vi "Create from SCP Receive.vi"(8 "Error In":errorcluster, 10 "Remote Source Path":string, 11 "Session":refnum<class "Session.lvclass">) -> (0 "Error Out":errorcluster, 2 "File Information":T3, 3 "Channel":refnum<class "Channel.lvclass">)   [LabVIEW 2021, in "Field_RnD_Services_LIBSSH2_Toolkit.lvlib" / "Channel.lvclass"]
doc: "Creates a new Channel object from a Session object but configured for downloading a file from a remote SSH server to the local machine."
uses:
  Channel.lvclass
  Session/Session.lvclass
  Type Definitions/Permissions.ctl
  Type Definitions/Modes.ctl
  Channel.lvclass/Channel.ctl
  File Info/Support/Create from Session.vi
  File Info/Support/Destroy to Channel.vi
  Field_RnD_Services_LIBSSH2_Toolkit.lvlib
  File Info/File Info.lvclass
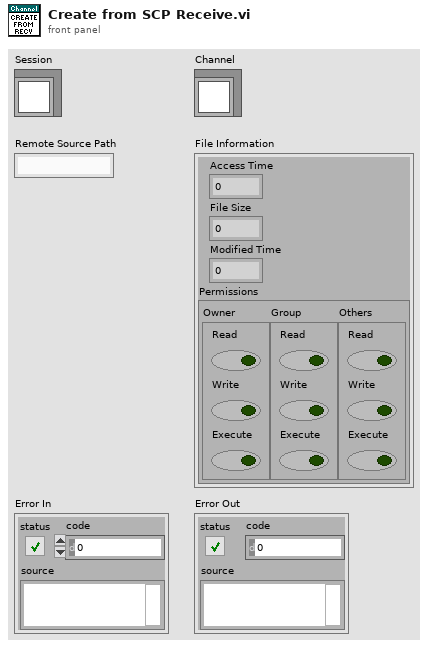
[diagram p1: front panel]
types:
  T1 = typedef "Field_RnD_Services_LIBSSH2_Toolkit.lvlib/Permissions.ctl" = cluster{"Owner":T2, "Group":T2, "Others":T2}
  T2 = typedef "Field_RnD_Services_LIBSSH2_Toolkit.lvlib/Modes.ctl" = cluster{"Read":bool, "Write":bool, "Execute":bool}
  T3 = cluster{"Access Time":u64, "File Size":u64, "Modified Time":u64, "Permissions":T1}
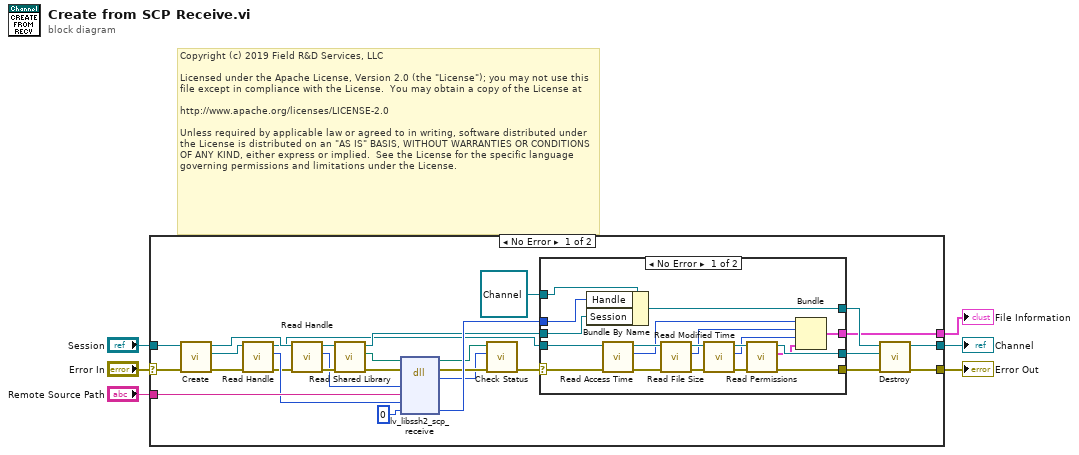
[diagram p0: block diagram]
diagram:
  # "Copyright (c) 2019 Field R&D Services, LLC\n\nLicensed under the Apache License, Version 2.0 (the \"License\"); you may not use this file except in compliance with the License.  You may obtain a copy of the License at\n\nhttp://www.apache.org/licenses/LICENSE-2.0\n\nUnless required by applicable law or agreed to in writing, software distributed under the License is distributed on an \"AS IS\" BASIS, WITHOUT WARRANTIES OR CONDITIONS OF ANY KIND, either express or implied.  See the License for the specific language governing permissions and limitations under the License."
  n1 = case shown="No Error" "Error In" {
    selector: "Error In" -> [w18 w57]
    tunnel: [w11 w57] -> w5
    tunnel: "Session" -> [w19 _]
    tunnel: [w13 _] -> w3
    tunnel: "Remote Source Path" -> [w21 _]
    tunnel: [w7 _] -> w1
    frame No Error {
      n2 = call-poly "Create.vi"("Error In"=w18, "Session In"=w19) -> ("Error Out"=w9:errorcluster, "File Info"=w8:refnum<class "File Info.lvclass">, "Session Out"=w17:refnum<class "Session.lvclass">)  [unwired: 7 in]
      n3 = call "Read Handle.vi"("Error In"=w9, "File Info In"=w8) -> ("Error Out"=w10:errorcluster, "Handle"=w20:u64, "File Info Out"=w16:refnum<class "File Info.lvclass">)  [unwired: 7 in]
      n4 = call "Read Handle.vi"("Error In"=w10, "Session In"=w17) -> ("Erorr Out"=w32:errorcluster, "Handle"=w29:u64, "Session Out"=w33:refnum<class "Session.lvclass">)  [unwired: 7 in]
      n5 = call "Read Shared Library.vi"("Error In"=w32, "Session In"=w33) -> ("Erorr Out"=w31:errorcluster, "libssh2lv Shared Library"=w30:path, "Session Out"=w22:refnum<class "Session.lvclass">)  [unwired: 7 in]
      n6 = dll-call lib="libssh2lv.*" fn="lv_libssh2_scp_receive"(path in=w30, error in=w31, "session"=w29, "path"=w21, "file_info"=w20, "handle"=u64 0) -> (path out=w24:path, error out=w26:errorcluster, "status"=w25:i32, "handle"=w27:u64)  [unwired: 4 in]
      n7 = call "Check Status.vi"("Error In"=w26, "Status"=w25, "libssh2lv Shared Library In"=w24) -> ("Error Out"=w23:errorcluster)  [unwired: 7 in, 1 out]
      n8 = case shown="No Error" w23 {
        selector: w23 -> [w41 w56]
        tunnel: [w50 w55] -> w14
        tunnel: w27 -> [w53 _]
        tunnel: [w40 w56] -> w12
        tunnel: w22 -> [w52 _]
        tunnel: refnum<class "Channel.lvclass"> refnum ("Toolkit.lvlib:Channel.lvclass") -> [w51 w55]
        tunnel: w16 -> [w43 w54]
        tunnel: [w42 w54] -> w15
        tunnel: [w35 _] -> w7
        frame No Error {
          n9 = Bundle By Name(cluster=w51, "Handle"=w53, "Session"=w52) -> (w50:refnum<class "Channel.lvclass">)
          n10 = call "Read Access Time.vi"("Error In"=w41, "File Info In"=w43) -> ("Error Out"=w48:errorcluster, "Access Time"=w39:u64, "File Info Out"=w49:refnum<class "File Info.lvclass">)  [unwired: 7 in]
          n11 = call "Read File Size.vi"("Error In"=w48, "File Info In"=w49) -> ("Error Out"=w46:errorcluster, "File Size"=w38:u64, "File Info Out"=w47:refnum<class "File Info.lvclass">)  [unwired: 7 in]
          n12 = call "Read Modified Time.vi"("Error In"=w46, "File Info In"=w47) -> ("Error Out"=w44:errorcluster, "Modified Time"=w37:u64, "File Info Out"=w45:refnum<class "File Info.lvclass">)  [unwired: 7 in]
          n13 = call "Read Permissions.vi"("Error In"=w44, "File Info In"=w45) -> ("Error Out"=w40:errorcluster, "Permissions"=w36:T1, "File Info Out"=w42:refnum<class "File Info.lvclass">)  [unwired: 7 in]
          n14 = Bundle("Access Time"=w39, "File Size"=w38, "Modified Time"=w37, "Permissions"=w36) -> (w35:T3)  [unwired: 1 in]
        }
        frame Error {
        }
      }
      n15 = call-poly "Destroy.vi"("Error In"=w12, "File Info"=w15, "Channel In"=w14) -> ("Error Out"=w11:errorcluster, "Channel Out"=w13:refnum<class "Channel.lvclass">)  [unwired: 7 in]
    }
    frame Error {
    }
  }
  "Error Out" <- w5
  "Channel" <- w3
  "File Information" <- w1
